vi "SetPower.vi"(7 "Sync Group":u8=1 format="%08b", 8 "error in (no error)":errorcluster, 10 "MotorPower":dbl(slide) scale=-1.0..1.0, 11 "DriveMotorsRight in":refnum<class "DriveMotorsRight.lvclass">) -> (0 "error out":errorcluster, 3 "DriveMotorsRight out":refnum<class "DriveMotorsRight.lvclass">)   [LabVIEW 2013, in "DriveMotorsRight.lvclass"]
uses:
  DriveMotorsRight.lvclass
  DriveMotors/DriveMotors.lvclass
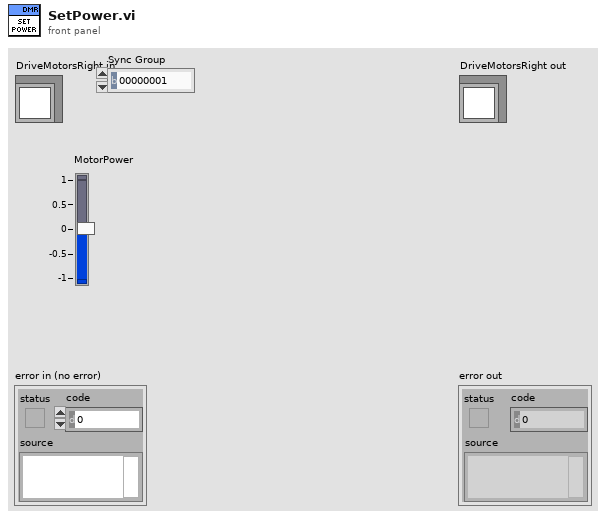
[diagram p1: front panel]
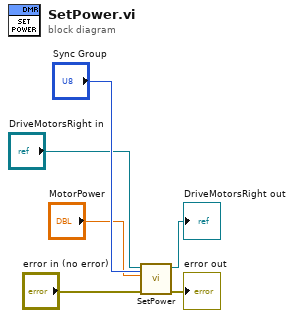
[diagram p0: block diagram]
diagram:
  n1 = call-parent "SetPower.vi"(7:"Sync Group", "error in (no error)"="error in (no error)", "MotorPower"="MotorPower", "DriveMotors in"="DriveMotorsRight in") -> ("error out"=→"error out":errorcluster, "DriveMotors out"=→"DriveMotorsRight out":refnum<class "DriveMotorsRight.lvclass">)  [unwired: 6 in]
